vi "Bead Tracking Overlay bead match.vi"(6 "Bead number":i32, 8 "error in (no error)":errorcluster, 9 "Y":dbl, 10 "X":dbl, 11 "Image":T1) -> (0 "error out":errorcluster, 3 "Image out":T1)   [LabVIEW 2011]
uses:
  <vilib>/vision/Image Controls.llb/IMAQ Image.ctl
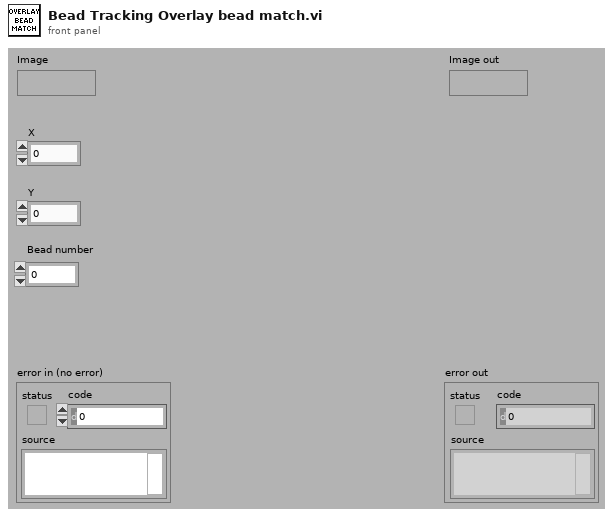
[diagram p1: front panel]
types:
  T1 = typedef "IMAQ Image.ctl" = refnum<image>
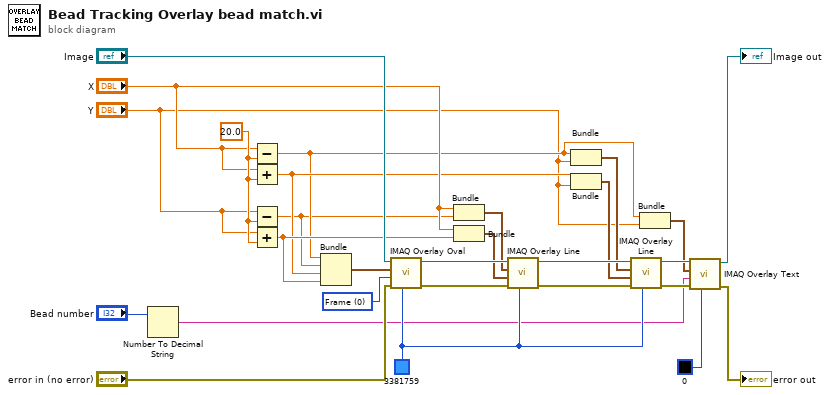
[diagram p0: block diagram]
diagram:
  w25 = u32 0 items=["Frame", "Fill"] ("Drawing Mode (Frame)")
  w19 = u32 3381759 ("Color")
  w24 = 20.0 ("y")
  n1 = Number To Decimal String(number="Bead number") -> (decimal integer string=w6:string)  [unwired: 1 in]
  n2 = Subtract(x="X", y=w24) -> (x-y=w4:dbl)
  n3 = Add(x="X", y=w24) -> (x+y=w14:dbl)
  n4 = Subtract(x="Y", y=w24) -> (x-y=w1:dbl)
  n5 = Add(x="Y", y=w24) -> (x+y=w15:dbl)
  n6 = Bundle(w4, w1, w14, w15) -> (w28:cluster{dbl, dbl, dbl, dbl})  [unwired: 1 in]
  n7 = call "IMAQ Overlay Oval"("Color"=w19, "error in (no error)"="error in (no error)", "Drawing Mode (Frame)"=w25, "Bounding Rectangle"=w28, "Image"="Image") -> ("error out"=w22:errorcluster, "Image Out"=w23:T1)  [unwired: 5 in]
  n8 = Bundle("X"="X", w1) -> (w17:cluster{"X":dbl, dbl})  [unwired: 1 in]
  n9 = Bundle("X"="X", w15) -> (w18:cluster{"X":dbl, dbl})  [unwired: 1 in]
  n10 = call "IMAQ Overlay Line"("Color"=w19, "error in (no error)"=w22, "End Point"=w18, "Start Point"=w17, "Image"=w23) -> ("error out"=w20:errorcluster, "Image Out"=w21:T1)  [unwired: 5 in]
  n11 = Bundle(w4, "Y"="Y") -> (w13:cluster{dbl, "Y":dbl})  [unwired: 1 in]
  n12 = Bundle(w14, "Y"="Y") -> (w12:cluster{dbl, "Y":dbl})  [unwired: 1 in]
  n13 = call "IMAQ Overlay Line"("Color"=w19, "error in (no error)"=w20, "End Point"=w12, "Start Point"=w13, "Image"=w21) -> ("error out"=w10:errorcluster, "Image Out"=w11:T1)  [unwired: 5 in]
  n14 = Bundle(w4, "Y"="Y") -> (w5:cluster{dbl, "Y":dbl})  [unwired: 1 in]
  n15 = call "IMAQ Overlay Text"("Text Color (black)"=u32 0, "error in (no error)"=w10, "String"=w6, "Origin"=w5, "Image"=w11) -> ("error out"=→"error out":errorcluster, "Image Out"=→"Image out":T1)  [unwired: 5 in]
